vi "Initialize Actor.vi"(7 "Host Name":string, 8 "error in (no error)":errorcluster, 9 "Actor Name":string, 10 "Message Broker Interface":refnum<class "Message Broker Interface.lvclass">, 11 "Car Wash Console in":refnum<class "Car Wash Console.lvclass">) -> (0 "error out":errorcluster, 3 "Car Wash Console out":refnum<class "Car Wash Console.lvclass">)   [LabVIEW 2016, in "CLD Exam - Car Wash.lvlib" / "Car Wash Console.lvclass"]
doc: "--\nCopyright © 2017 Composed SystemsI All rights reserved.\n\nAuthor: Jon McBee <jon.mcbee@composed.io>\n\nThis library is provided \"AS IS\" ,WITHOUT WARRANTIES OR\nCONDITIONS OF ANY KIND, either express or implied.\n\nComposed Systems -- composed.io\n\nStream 0.0.1.1\nJon McBee - Composed Systems\nCopyright (c) 2017, Composed Systems"
uses:
  Car Wash Console.lvclass
  Mediator/Classes/Message Broker Interface/Message Broker Interface.lvclass
  Car Wash Console.lvclass/Car Wash Console.ctl
  Mediator/Classes/Message Transport Event/Message Transport Event.lvclass
  D:/Repos/Stream/software/Mediator/Classes/Message Transport Interface/Message Transport Interface.lvclass
  Mediator/Classes/Mediated Synchronous Actor/Mediated Synchronous Actor.lvclass
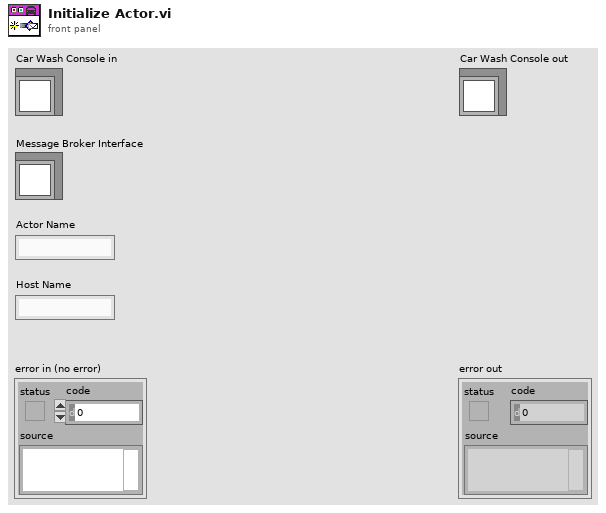
[diagram p1: front panel]
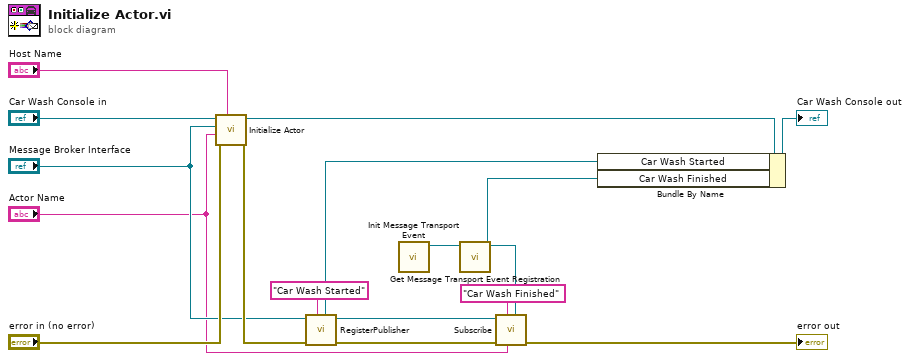
[diagram p0: block diagram]
diagram:
  n1 = call-parent "Initialize Actor.vi"("Host Name"="Host Name", "error in (no error)"="error in (no error)", "Actor Name"="Actor Name", "Message Broker Interface"="Message Broker Interface", "Mediated Synchronous Actor in"="Car Wash Console in") -> ("error out"=w12:errorcluster, "Mediated Synchronous Actor out"=w14:refnum<class "Car Wash Console.lvclass">)  [unwired: 5 in]
  n2 = call-dynamic "RegisterPublisher.vi"("Topic Name"="Car Wash Started", "error in (no error)"=w12, "Message Broker Interface in"="Message Broker Interface") -> ("error out"=w8:errorcluster, "Message Broker Interface out"=w5:refnum<class "Message Broker Interface.lvclass">, "Transport"=w9:refnum<class "Message Transport Queue.lvclass">)  [unwired: 4 in, 2 out]
  n3 = call "Init Message Transport Event.vi"() -> ("Message Transport Event out"=w4:refnum<class "Message Transport Event.lvclass">)  [unwired: 10 in, 1 out]
  n4 = call "Get Message Transport Event Registration.vi"("Message Transport Event in"=w4) -> ("Event Registration Refnum"=w1:refnum<event-registration>, "Message Transport Event out"=w2:refnum<class "Message Transport Event.lvclass">)  [unwired: 7 in, 2 out]
  n5 = call-dynamic "Subscribe.vi"("Message Transport Interface"=w2, "Subscriber Name"="Actor Name", "Topic Name"="Car Wash Finished", "error in (no error)"=w8, "Message Broker Interface in"=w5) -> ("error out"=→"error out":errorcluster)  [unwired: 4 in, 2 out]
  n6 = Bundle By Name(cluster=w14, "Car Wash Started"=w9, "Car Wash Finished"=w1) -> (→"Car Wash Console out":refnum<class "Car Wash Console.lvclass">)
